vi "Dashboard Main.vi"() -> ()   [LabVIEW 2012]
uses:
  Sally_Framework_2013/AutoEnum.ctl
  Sally_Framework_2013/LauncherPresets.ctl
  Sally_Framework_2013/AutoInstructArray.ctl
  Sally_Framework_2013/AutoInstruction.ctl
  <vilib>/event_ctls.llb/eventvkey.ctl
  DBNameEnum.ctl
  <vilib>/Utility/config.llb/Read Key (String).vi
  <vilib>/Utility/config.llb/Read Key (I32).vi
  <vilib>/Utility/config.llb/Write Key (String).vi
  <vilib>/Utility/config.llb/Write Key (I32).vi
  <vilib>/Utility/config.llb/NI_LVConfig.lvlib
panel:
  out "Battery Value":dbl(slide) scale=0.0..14.0 scale format="%#_2e"
  out "Battery":sgl(graph)
  in  "Camera Settings":T1={"Frate Rate"=30, "Compression"=30, "Size"=1} {"Frate Rate" scale=1.0..30.0; "Size" items=["640x480", "320x240", "160x120"]}
  out "Mode":T2(ring)=enum."Auto Disabled"
  out "Camera IP":string
  out "Robot IP":string
  in  "Dashboard Tab":T3(tab)
  in  "Use2DriveAlign":bool=TRUE
  out "DriveAlignLSRight":bool
  out "ClimbLS":bool
  in  "UseLauncherPID":bool=TRUE
  in  "UseAngleEncoder":bool=TRUE
  in  "UseLauncherEncoder":bool=TRUE
  out "LauncherAngleMatches":bool
  out "sDriveDistance":dbl
  out "Drive Loop Timing (ms)":u32
  in  "AutoEnum":T4=enum."BehindPyramid"
  out "LauncherMotorValue":dbl
  out "Version":string
  out "LauncherAngle":cluster{dbl, dbl}(knob) scale=0.0..55.0 scale format="%#2_3g"
  out "DriveAlignLSLeft":bool
  out "LauncherRPM":cluster{dbl, dbl}(knob) scale=0.0..4000.0
  in  "Disabled":T5=[{"Distance/Angle"=10.0, "Speed"=0.0, "Action"=enum."Wait", "NumFrisbees"=0}]
  in  "BehindPyramid":T5=[{"Distance/Angle"=30.0, "Speed"=2390.0, "Action"=enum."Aim", "NumFrisbees"=0}, {"Distance/Angle"=5.0, "Speed"=0.0, "Action"=enum."Wait", "NumFrisbees"=0}, {"Distance/Angle"=0.0, "Speed"=0.0, "Action"=enum."Shoot", "NumFrisbees"=4}]
  in  "CloseLeft":T5=[{"Distance/Angle"=34.0, "Speed"=2390.0, "Action"=enum."Aim", "NumFrisbees"=0}, {"Distance/Angle"=5.0, "Speed"=0.0, "Action"=enum."Wait", "NumFrisbees"=0}, {"Distance/Angle"=0.0, "Speed"=0.0, "Action"=enum."Shoot", "NumFrisbees"=4}]
  in  "CloseRight":T5=[{"Distance/Angle"=34.0, "Speed"=2390.0, "Action"=enum."Aim", "NumFrisbees"=0}, {"Distance/Angle"=5.0, "Speed"=0.0, "Action"=enum."Wait", "NumFrisbees"=0}, {"Distance/Angle"=0.0, "Speed"=0.0, "Action"=enum."Shoot", "NumFrisbees"=4}]
  in  "BackLeft":T5=[{"Distance/Angle"=29.0, "Speed"=2390.0, "Action"=enum."Aim", "NumFrisbees"=0}, {"Distance/Angle"=5.0, "Speed"=0.0, "Action"=enum."Wait", "NumFrisbees"=0}, {"Distance/Angle"=0.0, "Speed"=0.0, "Action"=enum."Shoot", "NumFrisbees"=4}]
  in  "BackRight":T5=[{"Distance/Angle"=29.0, "Speed"=2390.0, "Action"=enum."Aim", "NumFrisbees"=0}, {"Distance/Angle"=5.0, "Speed"=0.0, "Action"=enum."Wait", "NumFrisbees"=0}, {"Distance/Angle"=0.0, "Speed"=0.0, "Action"=enum."Shoot", "NumFrisbees"=4}]
  in  "BackupAuto":dbl[](array[numeric])=[2390.0, 30.0, 5.0, 4.0]
  in  "UseClusterArray":bool
  in  "PullbackTol":dbl=100.0
  in  "FireTol":dbl=10.0
  in  "LauncherRPMTol":dbl=10.0
  in  "LauncherAngleTol":dbl=0.05
  in  "InitialWait (ms)":dbl
  in  "WaitBetweenLaunch (ms)":dbl=1200.0
  in  "QSWaitBeforeFire (ms)":dbl=400.0
  in  "QSWaitBeforeRetract (ms)":dbl=100.0
  in  "AngleForwardValue":dbl=0.8
  in  "AngleBackwardValue":dbl=-0.8
  in  "RPMPresets":T7={"cPresetPyramid"=2390.0, "cPresetShort"=2390.0, "cPresetMid"=1950.0, "cPresetFar"=2390.0, "cPresetClimbHigh"=0.0, "cPresetClimbLow"=0.0}
  in  "AnglePresets":T7={"cPresetPyramid"=30.0, "cPresetShort"=50.0, "cPresetMid"=51.5, "cPresetFar"=25.0, "cPresetClimbHigh"=32.0, "cPresetClimbLow"=20.0}
  in  "Slider":dbl(slide) scale=0.0..100.0 scale format="%#_3g"
  in  "On/Off":bool caption="Solenoid"
  in  "Test Name":u16(ring) items=["Select the test to run...", "Example Test", "-------------------------------", "List of tests is built in robot code.", "Replace with your own automated tests."]
  in  "Test Tree":string(tree)
  in  "Motor":cluster{"Value":dbl, "Enable":bool} {"Value" scale=-1.0..1.0 scale format="%#_3g"}
  out "Progress":T8 {"Test Progress" scale=0.0..100.0}
  in  "Rev/Fwd":cluster{"Forward":bool, "Reverse":bool}
  in  "Ring":u16(ring) items=["Auto", "Fixed indoor", "Fixed outdoor 1", "Fixed outdoor 2", "Fixed fluorescent 1", "Fixed fluorescent 2", "Hold current"]
  in  "Listbox":i32(listbox)=8
  in  "Viewer":T9(tab)
  out "Mbps":dbl format="%#.1g"
  in  "Enable":bool=TRUE
  in  "DB Camera Config":bool
  out "Mbps":bool
  out "fps":dbl format="%#.1g"
  out "Image Error Message":string="Timeout in Camera Communications"
  out "Camera Image":T10(plugin-control)
  out "Buttons 1":cluster{"1":bool, "2":bool, "3":bool}
  out "Kinect 1":cluster{"X":dbl, "Y":dbl, "Z":dbl} {"X" scale=1.0..-1.0; "Y" scale=1.0..-1.0; "Z" scale=1.0..-1.0}
  out "Buttons 2":cluster{"1":bool, "2":bool, "3":bool}
  out "Kinect 2":cluster{"X":dbl, "Y":dbl, "Z":dbl} {"X" scale=1.0..-1.0; "Y" scale=1.0..-1.0; "Z" scale=1.0..-1.0}
  out "Version":string
  out "Skeleton Picture":picture
  out "Players":i8
  out "Tree":string(tree)
  # "Drive & Motors"
  # "Robot IP:"
  # "sLauncherRPM"
  # "TargetLauncherRPM"
  # "sLauncherAngle"
  # "LauncherTargetAngle"
  # "RPM\nAngle\nWait\nShootNum"
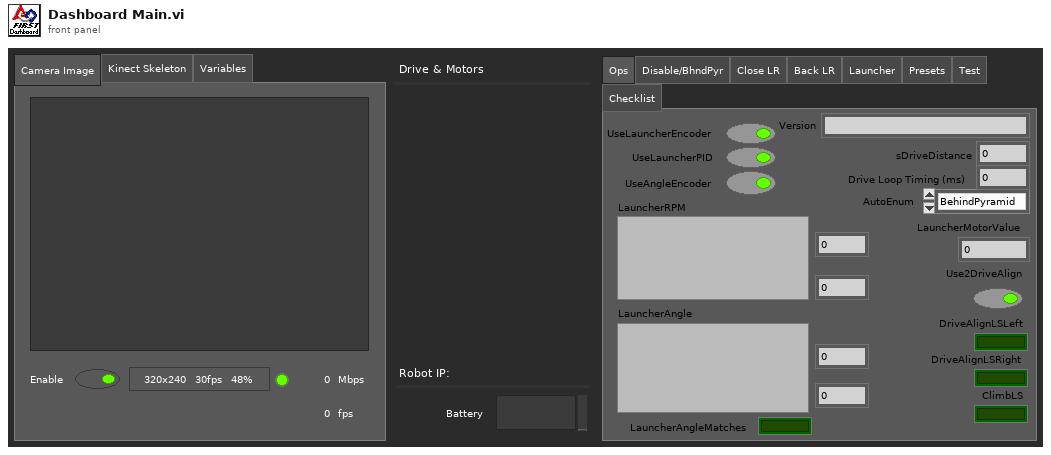
[diagram p1: front panel]
types:
  T1 = cluster{"Frate Rate":i32, "Compression":i32, "Size":u16}
  T2 = enum8{"Tele-Op Disabled", "Tele-Op Enabled", "Auto Disabled", "Auto Enabled", "Test Disabled", "Test Enabled", ""}
  T3 = enum32{"Ops", "Disable/BhndPyr", "Close LR", "Back LR", "Launcher", "Presets", "Test", "Checklist"}
  T4 = typedef "AutoEnum.ctl" = enum16{"Disabled", "BackRight", "BackLeft", "CloseRight", "CloseLeft", "BehindPyramid"}
  T5 = typedef "AutoInstructArray.ctl" = T6[]
  T6 = typedef "AutoInstruction.ctl" = cluster{"Distance/Angle":dbl, "Speed":dbl, "Action":enum16{"DriveForward", "Turn", "Aim", "Shoot", "Wait"}, "NumFrisbees":i32}
  T7 = typedef "LauncherPresets.ctl" = cluster{"cPresetPyramid":dbl, "cPresetShort":dbl, "cPresetMid":dbl, "cPresetFar":dbl, "cPresetClimbHigh":dbl, "cPresetClimbLow":dbl}
  T8 = cluster{"Test Progress":u8, "Test Progress Text":string}
  T9 = enum32{"Camera Image", "Kinect Skeleton", "Variables"}
  T10 = typedef "IMAQ Image.ctl" = refnum<image>
  T11 = typedef "Image Type" = u32
  T12 = typedef "LVBoundsTypeDef.ctl" = cluster{"Width":u32, "Height":u32}
  T13 = typedef "SkeletonTrackState.ctl" = enum32{"NotTracked", "PositionOnly", "Tracked"}
  T14 = cluster{"TrackingState":u8[], "Position":cluster{"x":sgl, "y":sgl, "z":sgl}, cluster{"x":sgl, "y":sgl, "z":sgl, sgl}[], "TrackState":T13}
  T15 = cluster{cluster{"ScaledToPercentRange":dbl, "ScaledToPercentRange":dbl, "ScaledToPercentRange":dbl}, cluster{bool, bool, bool}}[]
  T16 = cluster{cluster{"ScaledToPercentRange":dbl, "ScaledToPercentRange":dbl, "ScaledToPercentRange":dbl}, cluster{bool, bool, bool}}
  T17 = cluster{"ScaledToPercentRange":dbl, "ScaledToPercentRange":dbl, "ScaledToPercentRange":dbl}
  T18 = typedef "LVRectTypeDef.ctl" = cluster{"Left":i16, "Top":i16, "Right":i16, "Bottom":i16}
  T19 = typedef "DBNameEnum.ctl" = enum16{"AutoInstructions", "DriveLoopTime", "DriveAlignLSLeft", "DriveAlignLSRight", "Use2DriveAlign", "ClimbLS", "LauncherAngleMatches", "FrameworkVersion", "sLauncherAngle", "LauncherTargetAngle", "sLauncherRPM", "LauncherTargetRPM", "sDriveDistance", "LauncherMotorValue", "PullbackTol", "FireTol", "LauncherRPMTol", "LauncherAngleTol", "InitialWait", "WaitBetweenLaunch", "AnglePresets", "RPMPresets", "UseAngleEncoder", "UseLauncherEncoder", "UseLauncherPID", "QSWaitBeforeFire", "QSWaitBeforeRetract", "AngleForwardValue", "AngleBackwardValue", "UseClusterArray", "BackupAuto"}
  T20 = cluster{"Competition mode":bool, "Robot Link":bool, "Autonomous":bool, "Enabled":bool, "E-Stop":bool, "Simulated":bool, "TestMode":bool, "Docked Window":bool}
  T21 = typedef "NI_LVConfig.lvlib/Config Data RefNum.ctl" = refnum<k1>
  T22 = typedef "eventvkey.ctl" = enum16{"ASCII", "Enter", "Return", "Shift", "Ctrl", "Alt", "Cmd", "Opt", "Caps", "NumLock", "Clear", "Break", "Up", "Down", "Left", "Right", "Insert", "Delete", "Home", "End", "PageUp", "PageDown", "Escape", "Help", "Pause", "ScrollLock", "F1", "F2", "F3", "F4", "F5", "F6", "F7", "F8", "F9", "F10", "F11", "F12", "F13", "F14", "F15", "F16", "F17", "F18", "F19", "F20", "F21", "F22", "F23", "F24", "Play", "VolumeUp", "VolumeDown", "Mute", "Two Byte Char"}
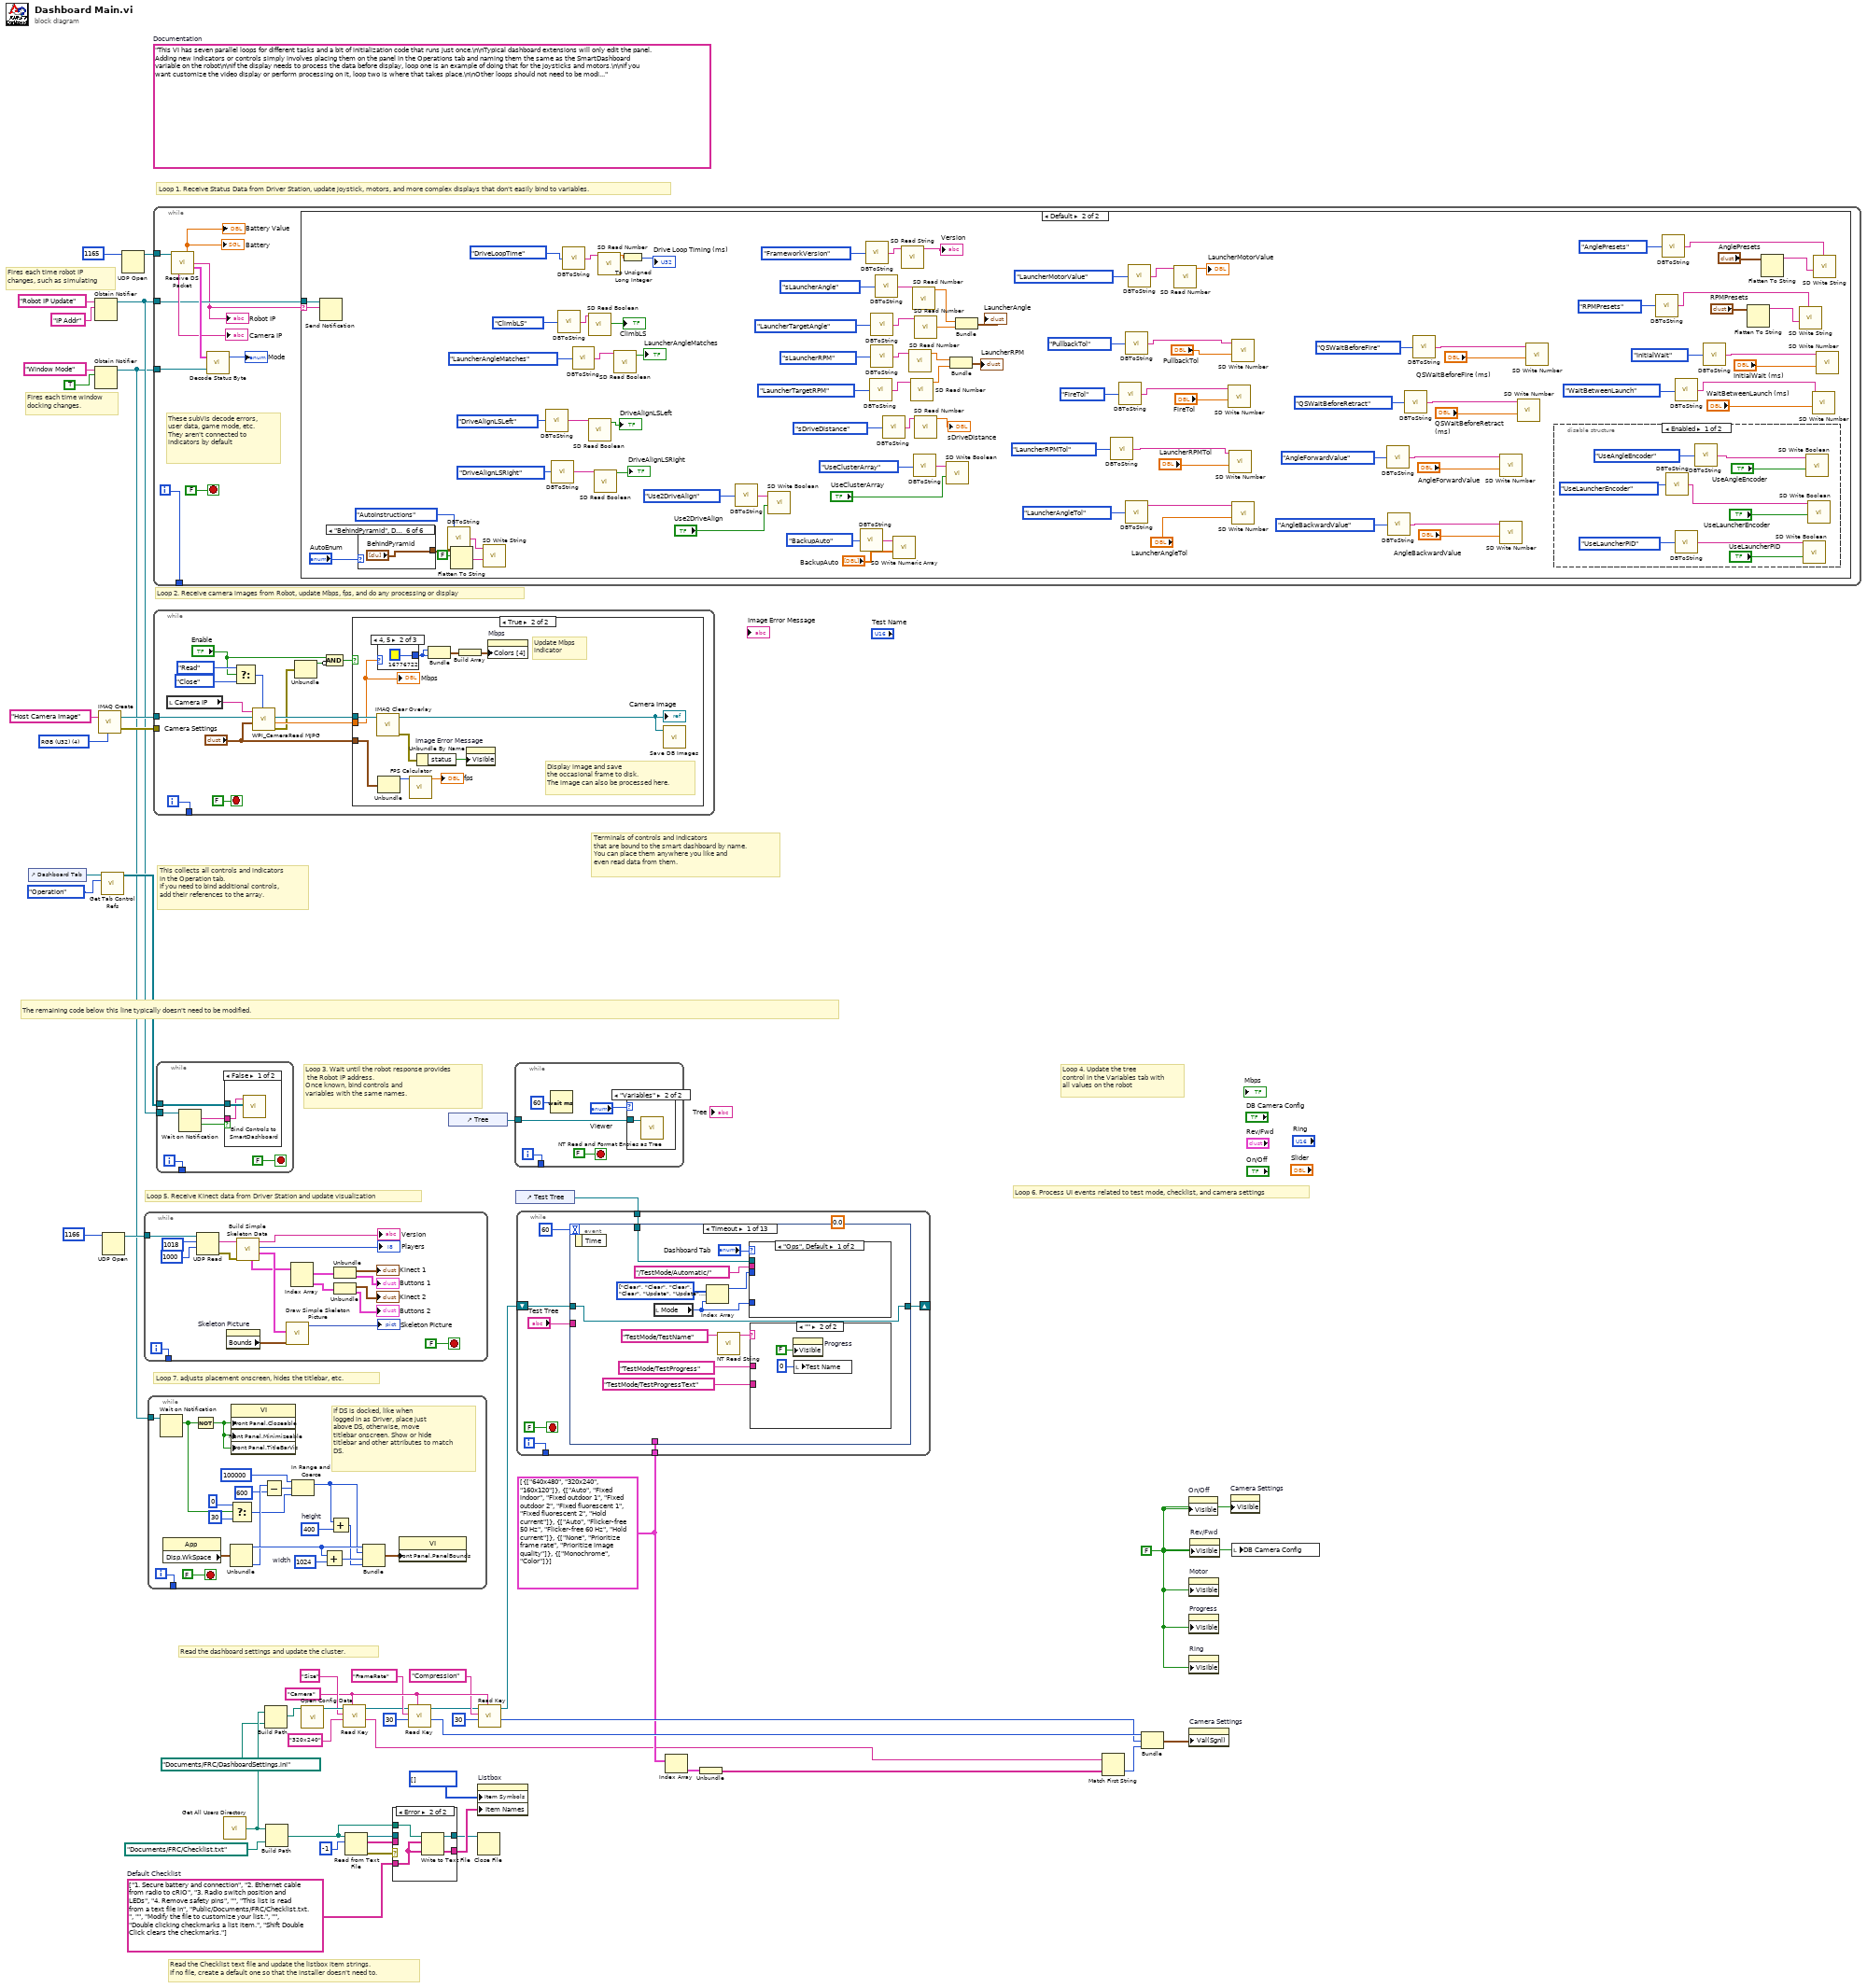
[diagram p0: block diagram]
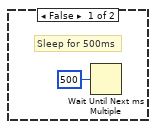
[diagram p3: hidden frame]
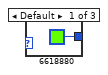
[diagram p4: hidden frame]
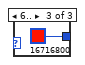
[diagram p5: hidden frame]
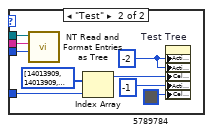
[diagram p7: hidden frame]
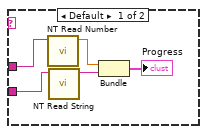
[diagram p8: hidden frame]
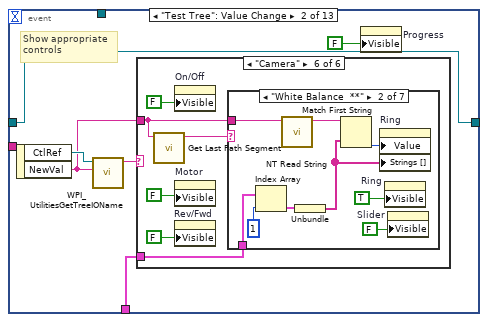
[diagram p9: hidden frame]
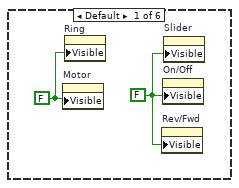
[diagram p10: hidden frame]
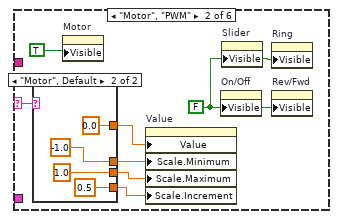
[diagram p11: hidden frame]
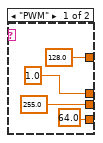
[diagram p12: hidden frame]
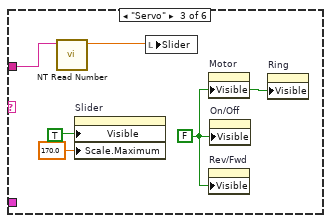
[diagram p13: hidden frame]
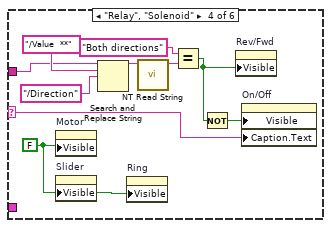
[diagram p14: hidden frame]
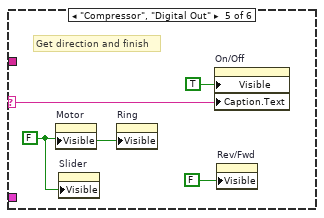
[diagram p15: hidden frame]
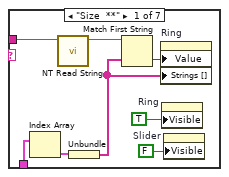
[diagram p16: hidden frame]
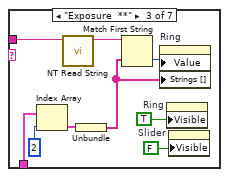
[diagram p17: hidden frame]
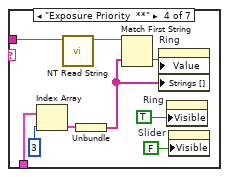
[diagram p18: hidden frame]
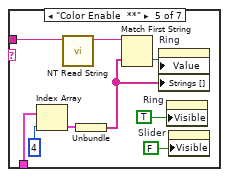
[diagram p19: hidden frame]
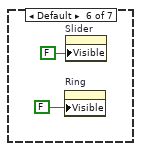
[diagram p20: hidden frame]
diagram:
  w21 = "Camera"
  w13 = cluster{string[]}[] [{["640x480", "320x240", "160x120"]}, {["Auto", "Fixed indoor", "Fixed outdoor 1", "Fixed outdoor 2", "Fixed fluorescent 1", "Fixed fluorescent 2", "Hold current"]}, {["Auto", "Flicker-free 50 Hz", "Flicker-free 60 Hz", "Hold current"]}, {["None", "Prioritize frame rate", "Prioritize image quality"]}, {["Monochrome", "Color"]}]
  w29 = string[] ["1. Secure battery and connection", "2. Ethernet cable from radio to cRIO", "3. Radio switch position and LEDs", "4. Remove safety pins", "", "This list is read from a text file in", "Public/Documents/FRC/Checklist.txt.", "", "Modify the file to customize your list.", "", "Double clicking checkmarks a list item.", "Shift Double Click clears the checkmarks."]  # Default Checklist
  w27 = FALSE ("Visible")
  (unwired) "This VI has seven parallel loops for different tasks and a bit of initialization code that runs just once.\n\nTypical dashboard extensions will only edit the panel. Adding new indicators or controls simply involves placing them on the panel in the Operations tab and naming them the same as the SmartDashboard variable on the robot\n\nIf the display needs to process the data before display, loop one is an example of doing that for the joysticks and motors.\n\nIf you want customize the video display or perform processing on it, loop two is where that takes place.\n\nOther loops should not need to be modified. They are pretty standard, and document the task they perform."  # Documentation
  w50 = T11 4 items=["Grayscale (U8)", "Grayscale (I16)", "Grayscale (SGL)", "Complex (CSG)", "RGB (U32)", "HSL (U32)", "RGB (U64)"] ("Image Type")
  # "Fires each time robot IP\nchanges, such as simulating"
  # "Fires each time window\ndocking changes."
  # "Read the Checklist text file and update the listbox item strings.\nIf no file, create a default one so that the installer doesn't need to."
  # "This collects all controls and indicators\nin the Operation tab.\nIf you need to bind additional controls,\nadd their references to the array."
  # "The remaining code below this line typically doesn't need to be modified."
  # "Loop 6. Process UI events related to test mode, checklist, and camera settings"
  # "Read the dashboard settings and update the cluster."
  # "Terminals of controls and indicators\nthat are bound to the smart dashboard by name.\nYou can place them anywhere you like and\neven read data from them."
  # "Loop 4. Update the tree\ncontrol in the Variables tab with\nall values on the robot"
  # "Loop 3. Wait until the robot response provides\n the Robot IP address.\nOnce known, bind controls and\nvariables with the same names."
  # "Loop 5. Receive Kinect data from Driver Station and update visualization"
  # "Loop 7. adjusts placement onscreen, hides the titlebar, etc."
  # "Loop 1. Receive Status Data from Driver Station, update joystick, motors, and more complex displays that don't easily bind to variables."
  # "Loop 2. Receive camera images from Robot, update Mbps, fps, and do any processing or display"
  n1 = control-ref of="Dashboard Tab"() -> (w43:refnum<vi>)
  n2 = Obtain Notifier(name (unnamed)="Robot IP Update", notification data type="IP Addr" ("name (unnamed)")) -> (notifier out=w40:refnum<notifier>)  [unwired: 2 in, 2 out]
  n3 = Obtain Notifier(name (unnamed)="Window Mode", notification data type=TRUE) -> (notifier out=w33:refnum<notifier>)  [unwired: 2 in, 2 out]
  n4 = call "IMAQ Create"("Image Name"="Host Camera Image", "Image Type"=w50) -> ("New Image"=w48:T10, "error out"=w47:errorcluster)  [unwired: 2 in, 1 out]
  n5 = call <vilib>:"Get Tab Control Refs.vi"("Page Index"=enum32{"Operation", "Test"}."Operation" ("Dashboard Tab"), "TabControl in"=w43) -> ("ControlsOnPage"=w44:refnum<vi>[])  [unwired: 9 in]
  n6 = UDP Open(11:u16 1166 ("port")) -> (port=w45:refnum<k16>)  [unwired: 2 in, 4 out]
  n7 = UDP Open(11:u16 1165 ("port")) -> (port=w51:refnum<k16>)  [unwired: 2 in, 4 out]
  n8 = while {
    tunnel: w45 -> [w69]
    tunnel: [w54] -> _
    i -> [w54]
    stop <- FALSE stop-if-true
    n9 = UDP Read(connection ID=w69, max size (548)=1018 ("bytes to read"), timeout ms (25000)=1000) -> (data out=w63:string, error out=w53:errorcluster)  [unwired: 1 in, 3 out]
    n10 = property on="Skeleton Picture" class="Pict"() -> ("Bounds"=w65:T12)  [unwired: 2 in, 2 out]
    n11 = call "Build Simple Skeleton Data.vi"("error in (no error)"=w53, "data in"=w63) -> ("Skeleton Data"=w64:T14, "NumPlayers"=→"Players":i8, "Version String"=→"Version":string, "Simple Joystick Info"=w61:T15)  [unwired: 5 in, 1 out]
    n12 = call "Draw Simple Skeleton Picture.vi"("Bounds"=w65, "Simple Skeleton"=w64) -> ("new picture out"=→"Skeleton Picture":picture)  [unwired: 9 in]
    n13 = Index Array(array=w61) -> (element #1=w60:T16, element #2=w59:T16)  [unwired: 2 in]
    n14 = Unbundle(w60) -> (→"Kinect 1":T17, →"Buttons 1":cluster{bool, bool, bool})
    n15 = Unbundle(w59) -> (→"Kinect 2":T17, →"Buttons 2":cluster{bool, bool, bool})
  }
  n16 = while {
    tunnel: w33 -> [w90]
    tunnel: [w88] -> _
    i -> [w88]
    stop <- FALSE stop-if-true
    w80 = 1024  # width
    w83 = 400  # height
    # "If DS is docked, like when\nlogged in as Driver, place just\nabove DS, otherwise, move\ntitlebar onscreen. Show or hide\ntitlebar and other attributes to match\nDS."
    n17 = Wait on Notification(notifier=w90) -> (notification=w75:bool)  [unwired: 3 in, 3 out]
    n18 = property class="App"() -> ("Disp.WkSpace"=w86:T18)  [unwired: 2 in, 2 out]
    n19 = Not(x=w75) -> (.not. x?=w89:bool)
    n20 = Unbundle(w86) -> ("Left"=w84:i16, "Bottom"=w81:i16)  [unwired: 2 out]
    n21 = Select(t=0, s=w75, f=30) -> (s? t:f=w74:i32)
    n22 = property class="VI"("Front Panel.Closeable"=w89, "Front Panel.Minimizeable"=w89, "Front Panel.TitleBarVis"=w89) -> ()  [unwired: 2 in, 2 out]
    n23 = Subtract(x=w81, y=600) -> (x-y=w78:i32)
    n24 = In Range and Coerce(upper limit=100000, x=w78, lower limit=w74) -> (coerced(x)=w72:i32)  [unwired: 1 out]
    n25 = Add(x=w84, y=w80) -> (x+y=w85:i32)
    n26 = Add(x=w72, y=w83) -> (x+y=w82:i32)
    n27 = Bundle("Left"=w84, w72, w85, w82) -> (w87:cluster{"Left":i16, i32, i32, i32})  [unwired: 1 out]
    n28 = property class="VI"("Front Panel.PanelBounds"=w87) -> ()  [unwired: 2 in, 2 out]
  }
  n29 = while {
    tunnel: w48 -> [w101]
    tunnel: w47 -> [_]
    tunnel: [w104] -> _
    i -> [w104]
    stop <- FALSE stop-if-true
    n30 = local read "Camera IP"() -> (w103:string)
    n31 = Select(t=enum16{"Read", "Reopen", "Close"}."Read" ("Operation"), s="Enable", f=enum16{"Read", "Reopen", "Close"}."Close" ("Operation")) -> (s? t:f=w96:enum16{"Read", "Reopen", "Close"})
    n32 = call <vilib>:"WPI_CameraRead MJPG.vi"("Operation"=w96, "Camera Settings"="Camera Settings", "Image"=w101, "address"=w103) -> ("error out"=w95:errorcluster, "Bandwidth (kbps)"=w99:dbl, "Image Out"=w100:T10)  [unwired: 5 in]
    n33 = Unbundle(w95) -> ("status"=w93:bool)  [unwired: 2 out]
    n34 = Compound Arithmetic op=AND("Enable", invert w93) -> (w92:bool)
    n35 = case shown="True" w92 {
      tunnel: "Camera Settings" -> [_ w108]
      tunnel: w100 -> [_ w111]
      tunnel: w99 -> [_ w110]
      frame False {
        # "Sleep for 500ms"
        n36 = Wait Until Next ms Multiple(millisecond multiple=u32 500) -> ()  [unwired: 1 out]
      }
      frame True {
        # "Display image and save\nthe occasional frame to disk.\nThe image can also be processed here."
        # "Update Mbps\nindicator"
        n37 = call "IMAQ Clear Overlay"("Image"=w111) -> ("error out"=w116:errorcluster, "Image Out"=w115:T10)  [unwired: 2 in, 7 out]
        "Camera Image" <- w115
        n38 = case shown="4, 5" w110 {
          tunnel: [u32 6618880 ("Color Box") u32 16776722 ("Color Box") u32 16716800 ("Color Box")] -> w112
          frame Default {
          }
          frame 4, 5 {
          }
          frame 6.. {
          }
        }
        n39 = Unbundle(w108) -> ("Frate Rate"=w107:i32)  [unwired: 2 out]
        n40 = call "FPS Calculator.vi"("Average Count"=w107) -> ("fps"=→"fps":dbl)  [unwired: 10 in]
        n41 = Unbundle By Name(w116) -> ("status"=w117:bool)
        n42 = Bundle("Color Box"=w112, "Color Box"=w112) -> (w114:cluster{"Color Box":u32, "Color Box":u32})  [unwired: 1 out]
        n43 = Build Array(w114) -> (w113:cluster{"Color Box":u32, "Color Box":u32}[])
        n44 = property on="Image Error Message" class="Str"("Visible"=w117) -> ()  [unwired: 2 in, 2 out]
        n45 = property on="Mbps" class="Bool (strict)"("Colors [4]"=w113) -> ()  [unwired: 2 in, 2 out]
        n46 = call "Save DB Images.vi"("Image"=w115) -> ()  [unwired: 2 in, 1 out]
        "Mbps" <- w110
      }
    }
  }
  n47 = while {
    tunnel: w51 -> [w128]
    tunnel: w40 -> [w122]
    tunnel: w33 -> [w126]
    tunnel: [w123] -> _
    i -> [w123]
    stop <- FALSE stop-if-true
    # "These subVIs decode errors, user data, game mode, etc.\nThey aren't connected to indicators by default"
    n48 = call "Receive DS Packet.vi"("Recv Socket"=w128) -> ("Battery"=→"Battery" →"Battery Value":sgl, "Robot IP Address"=w121:string, "Status"=w129:T20, "Camera IP Address"=→"Camera IP":string)  [unwired: 1 in, 10 out]
    "Robot IP" <- w121
    n49 = call "Decode Status Byte.vi"("Window Mode Notifier"=w126, "Status"=w129) -> ("Mode"=→"Mode":T2)  [unwired: 1 out]
    n50 = case shown="Default" w121 {
      selector: w121 -> [_ w223]
      tunnel: w122 -> [_ w224]
      frame "0.0.0.0" {
        # "Robot not responding, don't poll the variables"
      }
      frame Default {
        n51 = Send Notification(notification=w223, notifier=w224) -> ()  [unwired: 1 in, 2 out]
        n52 = case shown="\"BehindPyramid\", Default" "AutoEnum" {
          tunnel: ["Disabled" "BackRight" "BackLeft" "CloseRight" "CloseLeft" "BehindPyramid"] -> w158
          frame "Disabled" {
          }
          frame "BackRight" {
          }
          frame "BackLeft" {
          }
          frame "CloseRight" {
          }
          frame "CloseLeft" {
          }
          frame "BehindPyramid", Default {
          }
        }
        n53 = call "DBToString.vi"("Enum"=DBNameEnum."AutoInstructions") -> ("Refname"=w161:string)
        n54 = Flatten To String(anything=w158, prepend array or string size? (T)=FALSE) -> (data string=w159:string)  [unwired: 2 in, 2 out]
        n55 = call <vilib>:"SD Write String.vi"("String"=w159, "Name"=w161) -> ()  [unwired: 8 in, 2 out]
        n56 = call "DBToString.vi"("Enum"=DBNameEnum."DriveAlignLSLeft") -> ("Refname"=w167:string)
        n57 = call "DBToString.vi"("Enum"=DBNameEnum."DriveAlignLSRight") -> ("Refname"=w155:string)
        n58 = call "DBToString.vi"("Enum"=DBNameEnum."ClimbLS") -> ("Refname"=w164:string)
        n59 = call "DBToString.vi"("Enum"=DBNameEnum."DriveLoopTime") -> ("Refname"=w156:string)
        n60 = call "DBToString.vi"("Enum"=DBNameEnum."LauncherAngleMatches") -> ("Refname"=w163:string)
        n61 = call <vilib>:"SD Read Boolean.vi"("Name"=w164) -> ("Boolean"=→"ClimbLS":bool)  [unwired: 8 in, 2 out]
        n62 = call <vilib>:"SD Read Boolean.vi"("Name"=w167) -> ("Boolean"=→"DriveAlignLSLeft":bool)  [unwired: 8 in, 2 out]
        n63 = call <vilib>:"SD Read Boolean.vi"("Name"=w155) -> ("Boolean"=→"DriveAlignLSRight":bool)  [unwired: 8 in, 2 out]
        n64 = call <vilib>:"SD Read Number.vi"("Name"=w156) -> ("Numeric"=w222:dbl)  [unwired: 8 in, 2 out]
        n65 = call <vilib>:"SD Read Boolean.vi"("Name"=w163) -> ("Boolean"=→"LauncherAngleMatches":bool)  [unwired: 8 in, 2 out]
        n66 = To Unsigned Long Integer(number=w222) -> (unsigned 32bit integer=→"Drive Loop Timing (ms)":u32)
        n67 = call "DBToString.vi"("Enum"=DBNameEnum."Use2DriveAlign") -> ("Refname"=w151:string)
        n68 = call <vilib>:"SD Write Boolean.vi"("Boolean"="Use2DriveAlign", "Name"=w151) -> ()  [unwired: 8 in, 2 out]
        n69 = call "DBToString.vi"("Enum"=DBNameEnum."BackupAuto") -> ("Refname"=w133:string)
        n70 = call "DBToString.vi"("Enum"=DBNameEnum."FrameworkVersion") -> ("Refname"=w171:string)
        n71 = call "DBToString.vi"("Enum"=DBNameEnum."LauncherTargetRPM") -> ("Refname"=w172:string)
        n72 = call "DBToString.vi"("Enum"=DBNameEnum."LauncherTargetAngle") -> ("Refname"=w174:string)
        n73 = call "DBToString.vi"("Enum"=DBNameEnum."sLauncherRPM") -> ("Refname"=w173:string)
        n74 = call "DBToString.vi"("Enum"=DBNameEnum."sLauncherAngle") -> ("Refname"=w175:string)
        n75 = call "DBToString.vi"("Enum"=DBNameEnum."sDriveDistance") -> ("Refname"=w169:string)
        n76 = call <vilib>:"SD Write Numeric Array.vi"("Numeric Array"="BackupAuto", "Name"=w133) -> ()  [unwired: 8 in, 2 out]
        n77 = call <vilib>:"SD Read String.vi"("Name"=w171) -> ("String"=→"Version":string)  [unwired: 8 in, 2 out]
        n78 = call <vilib>:"SD Read Number.vi"("Name"=w173) -> ("Numeric"=w204:dbl)  [unwired: 8 in, 2 out]
        n79 = call <vilib>:"SD Read Number.vi"("Name"=w172) -> ("Numeric"=w205:dbl)  [unwired: 8 in, 2 out]
        n80 = call <vilib>:"SD Read Number.vi"("Name"=w175) -> ("Numeric"=w208:dbl)  [unwired: 8 in, 2 out]
        n81 = call "DBToString.vi"("Enum"=DBNameEnum."UseClusterArray") -> ("Refname"=w136:string)
        n82 = call <vilib>:"SD Read Number.vi"("Name"=w174) -> ("Numeric"=w209:dbl)  [unwired: 8 in, 2 out]
        n83 = call <vilib>:"SD Read Number.vi"("Name"=w169) -> ("Numeric"=→"sDriveDistance":dbl)  [unwired: 8 in, 2 out]
        n84 = call <vilib>:"SD Write Boolean.vi"("Boolean"="UseClusterArray", "Name"=w136) -> ()  [unwired: 8 in, 2 out]
        n85 = Bundle("Numeric"=w204, "Numeric"=w205) -> (→"LauncherRPM":cluster{"Numeric":dbl, "Numeric":dbl})  [unwired: 1 in]
        n86 = Bundle("Numeric"=w208, "Numeric"=w209) -> (→"LauncherAngle":cluster{"Numeric":dbl, "Numeric":dbl})  [unwired: 1 in]
        n87 = call "DBToString.vi"("Enum"=DBNameEnum."LauncherRPMTol") -> ("Refname"=w184:string)
        n88 = call "DBToString.vi"("Enum"=DBNameEnum."FireTol") -> ("Refname"=w183:string)
        n89 = call "DBToString.vi"("Enum"=DBNameEnum."PullbackTol") -> ("Refname"=w182:string)
        n90 = call "DBToString.vi"("Enum"=DBNameEnum."LauncherAngleTol") -> ("Refname"=w185:string)
        n91 = call "DBToString.vi"("Enum"=DBNameEnum."LauncherMotorValue") -> ("Refname"=w181:string)
        n92 = call <vilib>:"SD Read Number.vi"("Name"=w181) -> ("Numeric"=→"LauncherMotorValue":dbl)  [unwired: 8 in, 2 out]
        n93 = call <vilib>:"SD Write Number.vi"("Numeric"="FireTol", "Name"=w183) -> ()  [unwired: 8 in, 2 out]
        n94 = call <vilib>:"SD Write Number.vi"("Numeric"="LauncherRPMTol", "Name"=w184) -> ()  [unwired: 8 in, 2 out]
        n95 = call <vilib>:"SD Write Number.vi"("Numeric"="PullbackTol", "Name"=w182) -> ()  [unwired: 8 in, 2 out]
        n96 = call <vilib>:"SD Write Number.vi"("Numeric"="LauncherAngleTol", "Name"=w185) -> ()  [unwired: 8 in, 2 out]
        n97 = call "DBToString.vi"("Enum"=DBNameEnum."AngleForwardValue") -> ("Refname"=w141:string)
        n98 = call "DBToString.vi"("Enum"=DBNameEnum."AngleBackwardValue") -> ("Refname"=w138:string)
        n99 = call "DBToString.vi"("Enum"=DBNameEnum."QSWaitBeforeRetract") -> ("Refname"=w144:string)
        n100 = call "DBToString.vi"("Enum"=DBNameEnum."QSWaitBeforeFire") -> ("Refname"=w147:string)
        n101 = call <vilib>:"SD Write Number.vi"("Numeric"="AngleForwardValue", "Name"=w141) -> ()  [unwired: 8 in, 2 out]
        n102 = call <vilib>:"SD Write Number.vi"("Numeric"="AngleBackwardValue", "Name"=w138) -> ()  [unwired: 8 in, 2 out]
        n103 = call <vilib>:"SD Write Number.vi"("Numeric"="QSWaitBeforeRetract (ms)", "Name"=w144) -> ()  [unwired: 8 in, 2 out]
        n104 = call <vilib>:"SD Write Number.vi"("Numeric"="QSWaitBeforeFire (ms)", "Name"=w147) -> ()  [unwired: 8 in, 2 out]
        n105 = disable-structure shown="Enabled" {
          frame Enabled {
            n106 = call "DBToString.vi"("Enum"=DBNameEnum."UseLauncherEncoder") -> ("Refname"=w232:string)
            n107 = call "DBToString.vi"("Enum"=DBNameEnum."UseLauncherPID") -> ("Refname"=w231:string)
            n108 = call "DBToString.vi"("Enum"=DBNameEnum."UseAngleEncoder") -> ("Refname"=w236:string)
            n109 = call <vilib>:"SD Write Boolean.vi"("Boolean"="UseLauncherPID", "Name"=w231) -> ()  [unwired: 8 in, 2 out]
            n110 = call <vilib>:"SD Write Boolean.vi"("Boolean"="UseAngleEncoder", "Name"=w236) -> ()  [unwired: 8 in, 2 out]
            n111 = call <vilib>:"SD Write Boolean.vi"("Boolean"="UseLauncherEncoder", "Name"=w232) -> ()  [unwired: 8 in, 2 out]
          }
          frame Disabled {
          }
        }
        n112 = call "DBToString.vi"("Enum"=DBNameEnum."RPMPresets") -> ("Refname"=w192:string)
        n113 = call "DBToString.vi"("Enum"=DBNameEnum."AnglePresets") -> ("Refname"=w191:string)
        n114 = call "DBToString.vi"("Enum"=DBNameEnum."WaitBetweenLaunch") -> ("Refname"=w196:string)
        n115 = call "DBToString.vi"("Enum"=DBNameEnum."InitialWait") -> ("Refname"=w197:string)
        n116 = Flatten To String(anything="RPMPresets") -> (data string=w216:string)  [unwired: 3 in, 2 out]
        n117 = Flatten To String(anything="AnglePresets") -> (data string=w217:string)  [unwired: 3 in, 2 out]
        n118 = call <vilib>:"SD Write String.vi"("String"=w216, "Name"=w192) -> ()  [unwired: 8 in, 2 out]
        n119 = call <vilib>:"SD Write Number.vi"("Numeric"="WaitBetweenLaunch (ms)", "Name"=w196) -> ()  [unwired: 8 in, 2 out]
        n120 = call <vilib>:"SD Write String.vi"("String"=w217, "Name"=w191) -> ()  [unwired: 8 in, 2 out]
        n121 = call <vilib>:"SD Write Number.vi"("Numeric"="InitialWait (ms)", "Name"=w197) -> ()  [unwired: 8 in, 2 out]
      }
    }
  }
  n122 = while {
    tunnel: w44 -> [w245]
    tunnel: w40 -> [w242]
    tunnel: [w240] -> _
    i -> [w240]
    stop <- FALSE stop-if-true
    n123 = Wait on Notification(notifier=w242) -> (notification=w241:string, timed out?=w243:bool)  [unwired: 3 in, 2 out]
    n124 = case shown="False" w243 {
      tunnel: w245 -> [w247 _]
      tunnel: w241 -> [w246 _]
      frame False {
        n125 = call <vilib>:"Bind Controls to SmartDashboard.vi"("Bound Control Refs"=w247, "Server IP Address"=w246) -> ()  [unwired: 10 in]
      }
      frame True {
      }
    }
  }
  n126 = call "Get All Users Directory.vi"() -> ("All User Path"=w26:path)
  n127 = Build Path(base path=w26, name or relative path=path "Documents/FRC/DashboardSettings.ini") -> (appended path=w25:path)
  n128 = Build Path(base path=w26, name or relative path=path "Documents/FRC/Checklist.txt") -> (appended path=w30:path)
  n129 = call <vilib>:"Open Config Data.vi"("configuration file path"=w25) -> ("refnum"=w24:T21)  [unwired: 8 in, 2 out]
  n130 = call-poly <vilib>:"Read Key.vi"("section"=w21, "default value"="320x240", "key"="Size", "refnum"=w24) -> ("value"=w11:string, "refnum out"=w6:T21)  [unwired: 2 in, 4 out]
  n131 = Read from Text File(file (use dialog)=w30, count=-1 ("timeout ms (25000)")) -> (refnum out=w8:refnum<file>, text=w31:string[], error out=w32:errorcluster)  [unwired: 2 in, 1 out]
  n132 = case shown="Error" w32 {
    tunnel: w31 -> [w249 _]
    tunnel: [w249 w251] -> w28
    tunnel: w29 -> [_ w251]
    tunnel: w30 -> [_ w252]
    tunnel: [w248 w250] -> w7
    tunnel: w8 -> [w248 _]
    frame No Error {
    }
    frame Error {
      n133 = Write to Text File(file (use dialog)=w252, text=w251) -> (refnum out=w250:refnum<file>)  [unwired: 2 in, 2 out]
    }
  }
  n134 = call-poly <vilib>:"Read Key.vi"("section"=w21, "default value"=30, "key"="FrameRate", "refnum"=w6) -> ("value"=w16:i32, "refnum out"=w5:T21)  [unwired: 1 in, 5 out]
  n135 = control-ref of="Tree"() -> (w2:refnum<vi>)
  n136 = property on="Listbox" class="LstBox (strict)"("Item Symbols"=i32[] [], "Item Names"=w28) -> ()  [unwired: 2 in, 2 out]
  n137 = Close File(refnum=w7) -> ()  [unwired: 1 in, 2 out]
  n138 = call-poly <vilib>:"Read Key.vi"("section"=w21, "default value"=30, "key"="Compression", "refnum"=w5) -> ("value"=w15:i32, "refnum out"=w3:T21)  [unwired: 1 in, 5 out]
  n139 = while {
    tunnel: [w254] -> _
    tunnel: w2 -> [w253]
    i -> [w254]
    stop <- FALSE stop-if-true
    n140 = Wait (ms)(milliseconds to wait=u32 60) -> ()  [unwired: 1 out]
    n141 = case shown="\"Variables\"" "Viewer" {
      tunnel: w253 -> [_ w258]
      frame Default {
      }
      frame "Variables" {
        n142 = call <vilib>:"NT Read and Format Entries as Tree.vi"("Tree Refnum"=w258) -> ()  [unwired: 9 in, 2 out]
      }
    }
  }
  n143 = control-ref of="Test Tree"() -> (w1:refnum<vi>)
  n144 = while {
    tunnel: w13 -> [w263]
    shift-right: [w262] -> _
    shift-left: w3 -> [w261]
    tunnel: [w260] -> _
    tunnel: w1 -> [w259]
    i -> [w260]
    stop <- FALSE stop-if-true
    (unwired) 0.0 ("Meter")
    n145 = event shown="[0] Timeout" {
      selector: _ -> [_ _ _ _ _ _ _ _ _ _ _ _ _]
      dyn-events: _ -> [_ _ _ _ _ _ _ _ _ _ _ _ _]
      timeout: u32 60 ("milliseconds to wait") -> [_ _ _ _ _ _ _ _ _ _ _ _ _]
      tunnel: w259 -> [w273 _ _ _ _ _ _ _ _ _ _ _ _]
      tunnel: "Test Tree" -> [_ _ _ _ _ _ _ _ w467 w475 w477 w481 w489]
      tunnel: w263 -> [_ w295 _ _ _ _ w431 w461 _ _ _ _ _]
      tunnel: [w267 w294 _ w397 w405 w417 w430 w454 w466 w473 w476 w480 w488] -> w262
      tunnel: w261 -> [w267 w294 _ w397 w405 w417 w429 w454 w466 w473 w476 w480 w488]
      event Timeout {
        w272 = enum16{"Update", "Clear"}[] [enum."Clear", enum."Clear", enum."Clear", enum."Clear", enum."Update", enum."Update", enum."Clear"] items=["Update", "Clear"]
        n146 = event-data() -> ()  [unwired: 1 in, 1 out]
        n147 = local read "Mode"() -> (w270:T2)
        n148 = Index Array(array=w272, index=w270) -> (element=w271:enum16{"Update", "Clear"})
        n149 = call <vilib>:"NT Read String.vi"("Name"="TestMode/TestName") -> ("String"=w276:string)  [unwired: 9 in, 1 out]
        n150 = case shown="\"Ops\", Default" "Dashboard Tab" {
          tunnel: w273 -> [_ w286]
          tunnel: "/TestMode/Automatic/" ("Name Pattern") -> [_ w285]
          tunnel: w271 -> [_ w284]
          tunnel: w270 -> [_ w282]
          frame "Ops", Default {
          }
          frame "Test" {
            w281 = -2 ("Active Item:Row Number")
            n151 = call <vilib>:"NT Read and Format Entries as Tree.vi"("Operation"=w284, "Name Pattern"=w285, "Tree Refnum"=w286) -> ()  [unwired: 7 in, 2 out]
            n152 = Index Array(array=u32[] [14013909, 14013909, 14013909, 14013909, 14013909, 16777215, 14013909], index=w282) -> (element=w280:u32)
            n153 = property on="Test Tree" class="Tree (strict)"("Active Item Row Number"=w281, "ActiveColNum"=w281, "CellBG"=w280, "Active Item Row Number"=-1 ("Active Item:Row Number"), "CellBG"=u32 5789784 ("Color Box")) -> ()  [unwired: 2 in, 2 out]
          }
        }
        n154 = case shown="\"\"" w276 {
          tunnel: "TestMode/TestProgress" ("Name") -> [w288 _]
          tunnel: "TestMode/TestProgressText" ("Name") -> [w287 _]
          frame Default {
            n155 = call <vilib>:"NT Read Number.vi"("Name"=w288) -> ("Numeric"=w289:dbl)  [unwired: 9 in, 1 out]
            n156 = call <vilib>:"NT Read String.vi"("Name"=w287) -> ("String"=w290:string)  [unwired: 9 in, 1 out]
            n157 = Bundle("Numeric"=w289, "String"=w290) -> (→"Progress":cluster{"Numeric":dbl, "String":string})  [unwired: 1 in]
          }
          frame "" {
            n158 = property on="Progress" class="Clust (strict)"("Visible"=FALSE) -> ()  [unwired: 2 in, 2 out]
            n159 = local write "Test Name"(u16 0) -> ()
          }
        }
      }
      event "Test Tree": Value Change {
        # "Show appropriate\ncontrols"
        n160 = event-data() -> ("CtlRef"=w298:refnum<vi>, "NewVal"=w296:string)  [unwired: 1 in]
        n161 = call <vilib>:"WPI_UtilitiesGetTreeIOName.vi"("NewVal"=w296, "TreeControl in"=w298) -> ("I/O Name"=w299:string)  [unwired: 9 in]
        n162 = case shown="\"Camera\"" w299 {
          selector: w299 -> [_ w306 _ w324 w333 _]
          tunnel: w296 -> [_ _ w321 w323 _ w340]
          tunnel: w295 -> [_ _ _ _ _ w339]
          frame Default {
            w301 = FALSE ("Visible")
            w300 = FALSE ("Visible")
            n163 = property on="Motor" class="Clust (strict)"("Visible"=w300) -> ()  [unwired: 2 in, 2 out]
            n164 = property on="Ring" class="Ring (strict)"("Visible"=w300) -> ()  [unwired: 2 in, 2 out]
            n165 = property on="Rev/Fwd" class="Clust (strict)"("Visible"=w301) -> ()  [unwired: 2 in, 2 out]
            n166 = property on="On/Off" class="Bool (strict)"("Visible"=w301) -> ()  [unwired: 2 in, 2 out]
            n167 = property on="Slider" class="Slide (strict)"("Visible"=w301) -> ()  [unwired: 2 in, 2 out]
          }
          frame "Motor", "PWM" {
            w307 = FALSE ("Visible")
            n168 = case shown="\"Motor\", Default" w306 {
              tunnel: [1.0 ("Value") -1.0 ("Value")] -> w305
              tunnel: [255.0 ("Value") 1.0 ("Value")] -> w304
              tunnel: [128.0 ("Value") 0.0 ("Value")] -> w303
              tunnel: [64.0 ("Value") 0.5 ("Value")] -> w302
              frame "PWM" {
              }
              frame "Motor", Default {
              }
            }
            n169 = property on="Motor" class="Clust (strict)"("Visible"=TRUE) -> ()  [unwired: 2 in, 2 out]
            n170 = property on="Value" class="Slide (strict)"("Value"=w303, "Scale.Minimum"=w305, "Scale.Maximum"=w304, "Scale.Increment"=w302) -> ()  [unwired: 2 in, 2 out]
            n171 = property on="On/Off" class="Bool (strict)"("Visible"=w307) -> ()  [unwired: 2 in, 2 out]
            n172 = property on="Slider" class="Slide (strict)"("Visible"=w307) -> ()  [unwired: 2 in, 2 out]
            n173 = property on="Ring" class="Ring (strict)"("Visible"=w307) -> ()  [unwired: 2 in, 2 out]
            n174 = property on="Rev/Fwd" class="Clust (strict)"("Visible"=w307) -> ()  [unwired: 2 in, 2 out]
          }
          frame "Servo" {
            w319 = FALSE ("Visible")
            n175 = call <vilib>:"NT Read Number.vi"("Name"=w321) -> ("Numeric"=w320:dbl)  [unwired: 9 in, 1 out]
            n176 = property on="Slider" class="Slide (strict)"("Visible"=TRUE, "Scale.Maximum"=170.0 ("Scale.Range:Maximum")) -> ()  [unwired: 2 in, 2 out]
            n177 = local write "Slider"(w320) -> ()
            n178 = property on="Motor" class="Clust (strict)"("Visible"=w319) -> ()  [unwired: 2 in, 2 out]
            n179 = property on="Rev/Fwd" class="Clust (strict)"("Visible"=w319) -> ()  [unwired: 2 in, 2 out]
            n180 = property on="On/Off" class="Bool (strict)"("Visible"=w319) -> ()  [unwired: 2 in, 2 out]
            n181 = property on="Ring" class="Ring (strict)"("Visible"=w319) -> ()  [unwired: 2 in, 2 out]
          }
          frame "Relay", "Solenoid" {
            w322 = FALSE ("Visible")
            n182 = property on="Motor" class="Clust (strict)"("Visible"=w322) -> ()  [unwired: 2 in, 2 out]
            n183 = property on="Slider" class="Slide (strict)"("Visible"=w322) -> ()  [unwired: 2 in, 2 out]
            n184 = Search and Replace String(input string=w323, search string="/Value  **", replace string="/Direction") -> (result string=w329:string)  [unwired: 5 in, 3 out]
            n185 = property on="Ring" class="Ring (strict)"("Visible"=w322) -> ()  [unwired: 2 in, 2 out]
            n186 = call <vilib>:"NT Read String.vi"("Name"=w329) -> ("String"=w327:string)  [unwired: 9 in, 1 out]
            n187 = Equal?(x="Both directions", y=w327) -> (x = y?=w325:bool)
            n188 = Not(x=w325) -> (.not. x?=w326:bool)
            n189 = property on="Rev/Fwd" class="Clust (strict)"("Visible"=w325) -> ()  [unwired: 2 in, 2 out]
            n190 = property on="On/Off" class="Bool (strict)"("Visible"=w326, "Caption.Text"=w324) -> ()  [unwired: 2 in, 2 out]
          }
          frame "Compressor", "Digital Out" {
            w332 = FALSE ("Visible")
            # "Get direction and finish"
            n191 = property on="Motor" class="Clust (strict)"("Visible"=w332) -> ()  [unwired: 2 in, 2 out]
            n192 = property on="Slider" class="Slide (strict)"("Visible"=w332) -> ()  [unwired: 2 in, 2 out]
            n193 = property on="Ring" class="Ring (strict)"("Visible"=w332) -> ()  [unwired: 2 in, 2 out]
            n194 = property on="On/Off" class="Bool (strict)"("Visible"=TRUE, "Caption.Text"=w333) -> ()  [unwired: 2 in, 2 out]
            n195 = property on="Rev/Fwd" class="Clust (strict)"("Visible"=FALSE) -> ()  [unwired: 2 in, 2 out]
          }
          frame "Camera" {
            n196 = call <vilib>:"Get Last Path Segment.vi"("String in"=w340) -> ("String out"=w341:string)  [unwired: 10 in]
            n197 = property on="On/Off" class="Bool (strict)"("Visible"=FALSE) -> ()  [unwired: 2 in, 2 out]
            n198 = property on="Motor" class="Clust (strict)"("Visible"=FALSE) -> ()  [unwired: 2 in, 2 out]
            n199 = property on="Rev/Fwd" class="Clust (strict)"("Visible"=FALSE) -> ()  [unwired: 2 in, 2 out]
            n200 = case shown="\"White Balance  **\"" w341 {
              tunnel: w340 -> [w347 w356 w365 w374 w383 _ w389]
              tunnel: w339 -> [w345 w353 w362 w371 w380 _ _]
              frame "Size  **" {
                n201 = Index Array(array=w345) -> (element=w344:cluster{string[]})  [unwired: 1 in]
                n202 = call <vilib>:"NT Read String.vi"("Name"=w347) -> ("String"=w346:string)  [unwired: 9 in, 1 out]
                n203 = Unbundle(w344) -> (w342:string[])
                n204 = Match First String(2:w342, 3:w346) -> (0:w343:i32)  [unwired: 1 out]
                n205 = property on="Ring" class="Ring (strict)"("Value"=w343, "Strings []"=w342) -> ()  [unwired: 2 in, 2 out]
                n206 = property on="Ring" class="Ring (strict)"("Visible"=TRUE) -> ()  [unwired: 2 in, 2 out]
                n207 = property on="Slider" class="Slide (strict)"("Visible"=FALSE) -> ()  [unwired: 2 in, 2 out]
              }
              frame "White Balance  **" {
                n208 = Index Array(array=w353, index=1) -> (element=w354:cluster{string[]})
                n209 = call <vilib>:"NT Read String.vi"("Name"=w356) -> ("String"=w355:string)  [unwired: 9 in, 1 out]
                n210 = Unbundle(w354) -> (w351:string[])
                n211 = Match First String(2:w351, 3:w355) -> (0:w350:i32)  [unwired: 1 out]
                n212 = property on="Ring" class="Ring (strict)"("Value"=w350, "Strings []"=w351) -> ()  [unwired: 2 in, 2 out]
                n213 = property on="Ring" class="Ring (strict)"("Visible"=TRUE) -> ()  [unwired: 2 in, 2 out]
                n214 = property on="Slider" class="Slide (strict)"("Visible"=FALSE) -> ()  [unwired: 2 in, 2 out]
              }
              frame "Exposure  **" {
                n215 = Index Array(array=w362, index=2) -> (element=w363:cluster{string[]})
                n216 = call <vilib>:"NT Read String.vi"("Name"=w365) -> ("String"=w364:string)  [unwired: 9 in, 1 out]
                n217 = Unbundle(w363) -> (w359:string[])
                n218 = Match First String(2:w359, 3:w364) -> (0:w360:i32)  [unwired: 1 out]
                n219 = property on="Ring" class="Ring (strict)"("Value"=w360, "Strings []"=w359) -> ()  [unwired: 2 in, 2 out]
                n220 = property on="Ring" class="Ring (strict)"("Visible"=TRUE) -> ()  [unwired: 2 in, 2 out]
                n221 = property on="Slider" class="Slide (strict)"("Visible"=FALSE) -> ()  [unwired: 2 in, 2 out]
              }
              frame "Exposure Priority  **" {
                n222 = Index Array(array=w371, index=3) -> (element=w372:cluster{string[]})
                n223 = call <vilib>:"NT Read String.vi"("Name"=w374) -> ("String"=w373:string)  [unwired: 9 in, 1 out]
                n224 = Unbundle(w372) -> (w368:string[])
                n225 = Match First String(2:w368, 3:w373) -> (0:w369:i32)  [unwired: 1 out]
                n226 = property on="Ring" class="Ring (strict)"("Value"=w369, "Strings []"=w368) -> ()  [unwired: 2 in, 2 out]
                n227 = property on="Ring" class="Ring (strict)"("Visible"=TRUE) -> ()  [unwired: 2 in, 2 out]
                n228 = property on="Slider" class="Slide (strict)"("Visible"=FALSE) -> ()  [unwired: 2 in, 2 out]
              }
              frame "Color Enable  **" {
                n229 = Index Array(array=w380, index=4) -> (element=w381:cluster{string[]})
                n230 = call <vilib>:"NT Read String.vi"("Name"=w383) -> ("String"=w382:string)  [unwired: 9 in, 1 out]
                n231 = Unbundle(w381) -> (w377:string[])
                n232 = Match First String(2:w377, 3:w382) -> (0:w378:i32)  [unwired: 1 out]
                n233 = property on="Ring" class="Ring (strict)"("Value"=w378, "Strings []"=w377) -> ()  [unwired: 2 in, 2 out]
                n234 = property on="Ring" class="Ring (strict)"("Visible"=TRUE) -> ()  [unwired: 2 in, 2 out]
                n235 = property on="Slider" class="Slide (strict)"("Visible"=FALSE) -> ()  [unwired: 2 in, 2 out]
              }
              frame Default {
                n236 = property on="Ring" class="Ring (strict)"("Visible"=FALSE) -> ()  [unwired: 2 in, 2 out]
                n237 = property on="Slider" class="Slide (strict)"("Visible"=FALSE) -> ()  [unwired: 2 in, 2 out]
              }
              frame "Brightness  **", "Color Level  **", "Compression  **", "FPS  **", "Sharpness  **" {
                n238 = call <vilib>:"NT Read Number.vi"("Name"=w389) -> ("Numeric"=w388:dbl)  [unwired: 9 in, 1 out]
                n239 = local write "Slider"(w388) -> ()
                n240 = property on="Slider" class="Slide (strict)"("Visible"=TRUE, "Scale.Maximum"=100.0 ("Scale.Range:Maximum")) -> ()  [unwired: 2 in, 2 out]
                n241 = property on="Ring" class="Ring (strict)"("Visible"=FALSE) -> ()  [unwired: 2 in, 2 out]
              }
            }
          }
        }
        n242 = property on="Progress" class="Clust (strict)"("Visible"=FALSE) -> ()  [unwired: 2 in, 2 out]
      }
      event "Test Name": Mouse Enter {
        # "Populate the ring with the list of tests"
        n243 = event-data() -> ()  [unwired: 1 in, 1 out]
        n244 = call <vilib>:"NT Read String Array.vi"("Name"="TestMode/TestList") -> ("String Array"=w396:string[])  [unwired: 9 in, 1 out]
        n245 = Build Array (concatenate)("Select the test to run...", w396) -> (w395:string[])
        n246 = property on="Test Name" class="Ring (strict)"("Strings []"=w395) -> ()  [unwired: 2 in, 2 out]
      }
      event "Test Name": Value Change {
        w398 = FALSE ("Visible")
        # "Tell the robot the test name to run"
        n247 = event-data() -> ("NewVal"=w402:u16)  [unwired: 1 in]
        n248 = property on="Test Name" class="Ring (strict)"() -> ("Strings []"=w403:string[])  [unwired: 2 in, 2 out]
        n249 = local write "Progress"(T8 {"Test Progress"=0, "Test Progress Text"=""} ("Progress")) -> ()
        n250 = Index Array(array=w403, index=w402) -> (element=w401:string)
        n251 = call <vilib>:"NT Write String.vi"("String"=w401, "Name"="TestMode/TestName") -> ()  [unwired: 9 in, 1 out]
        n252 = property on="Progress" class="Clust (strict)"("Visible"=TRUE) -> ()  [unwired: 2 in, 2 out]
        n253 = property on="Motor" class="Clust (strict)"("Visible"=w398) -> ()  [unwired: 2 in, 2 out]
        n254 = property on="Slider" class="Slide (strict)"("Visible"=w398) -> ()  [unwired: 2 in, 2 out]
        n255 = property on="On/Off" class="Bool (strict)"("Visible"=w398) -> ()  [unwired: 2 in, 2 out]
        n256 = property on="Rev/Fwd" class="Clust (strict)"("Visible"=w398) -> ()  [unwired: 2 in, 2 out]
        n257 = property on="Ring" class="Ring (strict)"("Visible"=w398) -> ()  [unwired: 2 in, 2 out]
      }
      event "Listbox": Double Click {
        n258 = event-data() -> ("PlatMods.Shift"=w406:bool, "Row"=w408:i32)  [unwired: 1 in]
        n259 = case shown="False" w406 {
          tunnel: w408 -> [w412 _]
          tunnel: 1 -> [w411 _]
          frame False {
            n260 = property on="Listbox" class="LstBox (strict)"() -> ("Item Symbols"=w410:i32[])  [unwired: 2 in, 2 out]
            n261 = Replace Array Subset(array=w410, new element=w411, index=w412) -> (w409:i32[])
            n262 = property on="Listbox" class="LstBox (strict)"("Item Symbols"=w409) -> ()  [unwired: 2 in, 2 out]
          }
          frame True {
            w413 = 0 ("Top Row")
            n263 = property on="Listbox" class="LstBox (strict)"() -> ("Number of Rows"=w415:u32)  [unwired: 2 in, 2 out]
            n264 = Initialize Array(0, w415) -> (w414:i32[])
            n265 = property on="Listbox" class="LstBox (strict)"("Top Row"=w413, "Value"=w413, "Item Symbols"=w414) -> ()  [unwired: 2 in, 2 out]
          }
        }
      }
      event "Listbox": Key Down {
        n266 = event-data() -> ("VKey"=w419:T22)  [unwired: 1 in]
        n267 = case shown="\"Left\", \"Right\"" w419 {
          selector: w419 -> [w424 _]
          tunnel: eventvkey."Left" ("VKey") -> [w422 _]
          frame "Left", "Right" {
            n268 = Equal?(x=w422, y=w424) -> (x = y?=w423:bool)
            n269 = Select(t=0, s=w423, f=1) -> (s? t:f=w425:i32)
            n270 = property on="Listbox" class="LstBox (strict)"() -> ("Item Symbols"=w428:i32[])  [unwired: 2 in, 2 out]
            n271 = Replace Array Subset(array=w428, new element=w425, index="Listbox") -> (w427:i32[])
            n272 = property on="Listbox" class="LstBox (strict)"("Item Symbols"=w427) -> ()  [unwired: 2 in, 2 out]
          }
          frame Default {
          }
        }
      }
      event "DB Camera Config": Value Change {
        n273 = event-data() -> ("NewVal"=w432:bool)  [unwired: 1 in]
        n274 = case shown="False" w432 {
          tunnel: w431 -> [w441 _]
          tunnel: [w434 w452] -> w430
          tunnel: w429 -> [w433 w452]
          frame False {
            w448 = "Camera"
            w451 = FALSE ("Visible")
            n275 = local read "Camera Settings"() -> (w440:T1)
            n276 = Index Array(array=w441) -> (element=w444:cluster{string[]})  [unwired: 1 in]
            n277 = Unbundle(w440) -> ("Frate Rate"=w439:i32, "Compression"=w438:i32, "Size"=w442:u16)
            n278 = Unbundle(w444) -> (w443:string[])
            n279 = Index Array(array=w443, index=w442) -> (element=w437:string)
            n280 = call-poly <vilib>:"Write Key.vi"("section"=w448, "value"=w437, "key"="Size", "refnum"=w433) -> ("refnum out"=w450:T21)  [unwired: 2 in, 5 out]
            n281 = call-poly <vilib>:"Write Key.vi"("section"=w448, "value"=w439, "key"="FrameRate", "refnum"=w450) -> ("refnum out"=w449:T21)  [unwired: 1 in, 6 out]
            n282 = property on="Camera Settings" class="Clust (strict)"("Visible"=w451) -> ()  [unwired: 2 in, 2 out]
            n283 = local write "DB Camera Config"(w451) -> ()
            n284 = call-poly <vilib>:"Write Key.vi"("section"=w448, "value"=w438, "key"="Compression", "refnum"=w449) -> ("refnum out"=w435:T21)  [unwired: 1 in, 6 out]
            n285 = call <vilib>:"Close Config Data.vi"("refnum"=w435) -> ("file path"=w436:path)  [unwired: 2 in, 8 out]
            n286 = call <vilib>:"Open Config Data.vi"("configuration file path"=w436) -> ("refnum"=w434:T21)  [unwired: 8 in, 2 out]
          }
          frame True {
            n287 = property on="Camera Settings" class="Clust (strict)"("Visible"=TRUE) -> ()  [unwired: 2 in, 2 out]
          }
        }
      }
      event "Camera Settings": Value Change {
        n288 = event-data() -> ("NewVal"=w465:T1)  [unwired: 1 in]
        n289 = Index Array(array=w461) -> (element=w460:cluster{string[]})  [unwired: 1 in]
        n290 = Unbundle(w465) -> ("Frate Rate"=w456:i32, "Compression"=w455:i32, "Size"=w458:u16)
        n291 = Unbundle(w460) -> (w459:string[])
        n292 = Index Array(array=w459, index=w458) -> (element=w457:string)
        n293 = Format Into String(format string="%s   %dfps   %d%%", w457, w456, w455) -> (resulting string=w462:string)  [unwired: 2 in, 1 out]
        n294 = Build Array(w462) -> (w463:string[])
        n295 = property on="DB Camera Config" class="Bool (strict)"("Strings [4]"=w463) -> ()  [unwired: 2 in, 2 out]
      }
      event "Motor.Enable": Value Change {
        n296 = event-data() -> ("NewVal"=w471:bool)  [unwired: 1 in]
        n297 = Unbundle("Motor") -> ("Value"=w470:dbl)  [unwired: 1 out]
        n298 = Select(t=w470, s=w471, f=0.0) -> (s? t:f=w468:dbl)
        n299 = call <vilib>:"NT Write Number.vi"("Numeric"=w468, "Name"=w467) -> ()  [unwired: 9 in, 1 out]
      }
      event "Slider": Value Change {
        n300 = event-data() -> ("NewVal"=w474:dbl)  [unwired: 1 in]
        n301 = call <vilib>:"NT Write Number.vi"("Numeric"=w474, "Name"=w475) -> ()  [unwired: 9 in, 1 out]
      }
      event "On/Off": Value Change {
        n302 = event-data() -> ("NewVal"=w479:bool)  [unwired: 1 in]
        n303 = Boolean To (0,1)(Boolean=w479) -> (0, 1=w478:i16)
        n304 = call <vilib>:"NT Write Number.vi"("Numeric"=w478, "Name"=w477) -> ()  [unwired: 9 in, 1 out]
      }
      event "Rev/Fwd": Value Change {
        n305 = event-data() -> ("NewVal.Forward"=w487:bool, "NewVal.Reverse"=w486:bool)  [unwired: 1 in]
        n306 = Boolean To (0,1)(Boolean=w487) -> (0, 1=w483:i16)
        n307 = Boolean To (0,1)(Boolean=w486) -> (0, 1=w485:i16)
        n308 = Negate(x=w485) -> (-x=w484:i16)
        n309 = Add(x=w483, y=w484) -> (x+y=w482:i16)
        n310 = call <vilib>:"NT Write Number.vi"("Numeric"=w482, "Name"=w481) -> ()  [unwired: 9 in, 1 out]
      }
      event "Ring": Value Change {
        n311 = event-data() -> ("NewVal"=w491:u16)  [unwired: 1 in]
        n312 = property on="Ring" class="Ring (strict)"() -> ("Strings []"=w492:string[])  [unwired: 2 in, 2 out]
        n313 = Index Array(array=w492, index=w491) -> (element=w490:string)
        n314 = call <vilib>:"NT Write String.vi"("String"=w490, "Name"=w489) -> ()  [unwired: 9 in, 1 out]
      }
    }
  }
  n315 = Index Array(array=w13) -> (element=w14:cluster{string[]})  [unwired: 1 in]
  n316 = Unbundle(w14) -> (w12:string[])
  n317 = Match First String(2:w12, 3:w11) -> (0:w10:i32)  [unwired: 1 out]
  n318 = Bundle("value"=w16, "value"=w15, "index"=w10) -> (w4:cluster{"value":i32, "value":i32, "index":i32})  [unwired: 1 out]
  n319 = property on="On/Off" class="Bool (strict)"("Visible"=w27) -> ()  [unwired: 2 in, 2 out]
  n320 = property on="Motor" class="Clust (strict)"("Visible"=w27) -> ()  [unwired: 2 in, 2 out]
  n321 = property on="Progress" class="Clust (strict)"("Visible"=w27) -> ()  [unwired: 2 in, 2 out]
  n322 = property on="Ring" class="Ring (strict)"("Visible"=w27) -> ()  [unwired: 2 in, 2 out]
  n323 = property on="Camera Settings" class="Clust (strict)"("Val(Sgnl)"=w4) -> ()  [unwired: 2 in, 2 out]
  n324 = property on="Rev/Fwd" class="Clust (strict)"("Visible"=w27) -> ()  [unwired: 2 in, 2 out]
  n325 = property on="Camera Settings" class="Clust (strict)"("Visible"=w27) -> ()  [unwired: 2 in, 2 out]
  n326 = local write "DB Camera Config"(w27) -> ()
